vi "LoopThroughFrontPanelControls.vi"() -> ()   [LabVIEW 2019]
panel:
  out "Label.Text":string="all rows"
  in  "Numeric4":dbl
  in  "Numeric3":dbl
  in  "Numeric2":dbl
  in  "Numeric1":dbl
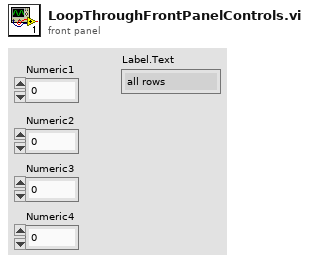
[diagram p1: front panel]
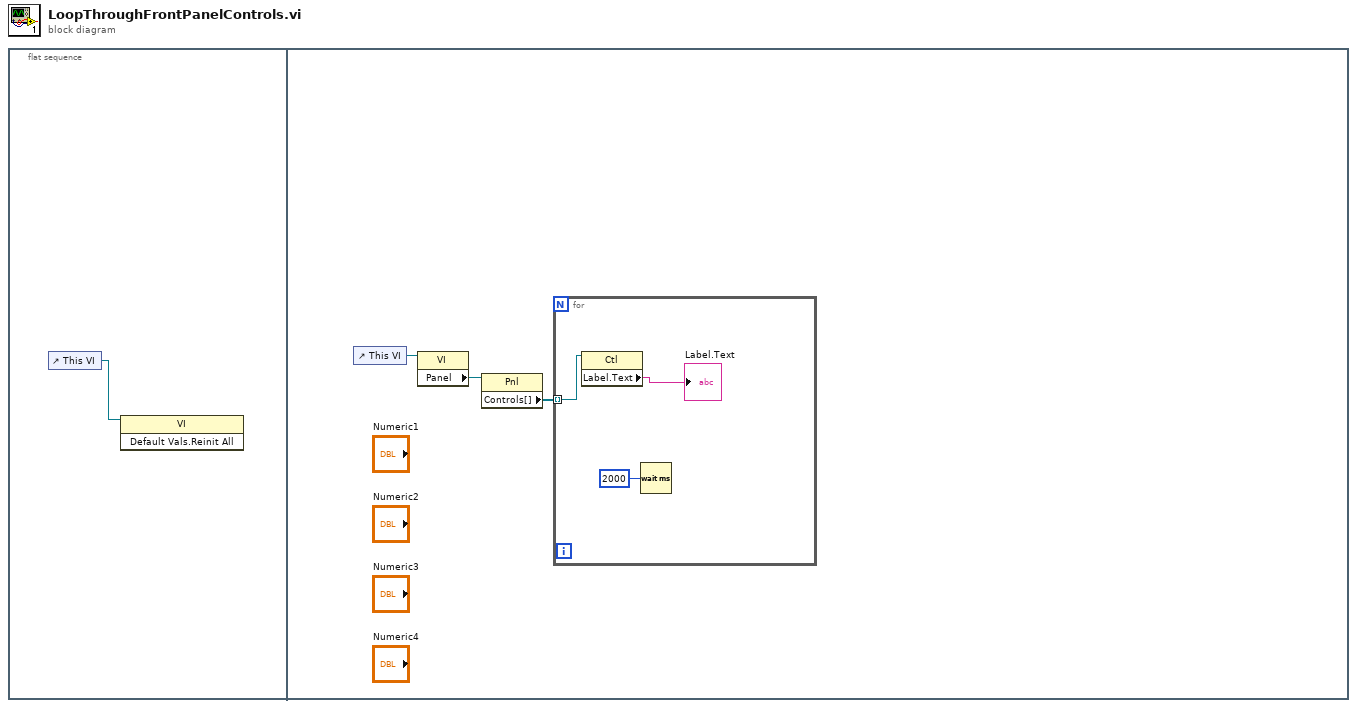
[diagram p0: block diagram]
diagram:
  n1 = flat-sequence {
    frame #0 {
      n2 = control-ref of="This VI"() -> (w1:refnum<vi>)
      n3 = invoke class="VI" method="Default Vals.Reinit All"(reference=w1) -> ()  [unwired: 2 in, 3 out]
    }
    frame #1 {
      n4 = control-ref of="This VI"() -> (w2:refnum<vi>)
      n5 = property class="VI"(reference=w2) -> ("Panel"=w3:refnum<vi>)  [unwired: 1 in, 2 out]
      n6 = property class="Pnl"(reference=w3) -> ("Controls[]"=w4:refnum<vi>[])  [unwired: 1 in, 2 out]
      n7 = for {
        tunnel: w4 -> [w5] mode=indexing
        n8 = property class="Ctl"(reference=w5) -> ("Label.Text"=→"Label.Text":string)  [unwired: 1 in, 2 out]
        n9 = Wait (ms)(milliseconds to wait=u32 2000) -> ()  [unwired: 1 out]
      }
    }
  }
